vi "Tuning Model - Trial and Error.vi"() -> ()   [LabVIEW 2021]
uses:
  <vilib>/Simulation/Scripting/Companion Diagram/SimConfigNode/SimParams.ctl
  <vilib>/Simulation/Scripting/Companion Diagram/SimConfigNode/_simSolvers.ctl
  <vilib>/Simulation/Implementation/Shared/SIMSCR Execution Mode.ctl
  <vilib>/Simulation/Param Hierarchy/Typedefs/SIMPH Param Control Actions.ctl
  <vilib>/Simulation/Implementation/Shared/NILVSim_ParamChanged.vi
  <vilib>/Simulation/Implementation/Shared/NILVSIM_BeginStep.vi
  <vilib>/Simulation/Implementation/Shared/NILVSim_Manager.vi
  <vilib>/Utility/error.llb/Clear Errors.vi
  <vilib>/Simulation/Implementation/Shared/NILVSim_FinalizeModel.vi
  <vilib>/Simulation/Implementation/Shared/SIM Unbundle Sim Info.vi
  <vilib>/Simulation/Implementation/Shared/NILVSim_Initialize.vi
  <vilib>/Simulation/Utility/Implementation/NILVSim Get Time and IsAcceptedStep.vi
  <vilib>/Simulation/Implementation/Shared/SIMSH Read Queue.vi
  <vilib>/Simulation/Implementation/Shared/NILVSim_GetModelError.vi
  <vilib>/Simulation/Implementation/Shared/SIM Bundle Sim Info.vi
  <vilib>/Simulation/Implementation/XNodeFramework/SimXNode/SimX.xnode
  Blackbox/Air Heater Black Box Model.vi
  <vilib>/Simulation/Scripting/Companion Diagram/SimConfigNode/SimDog.xnode
  SubVIs/Air Heater Model.vi
  <vilib>/Simulation/Implementation/Shared/NI_SIM_Implementation.lvlib
panel:
  out "Error [°C]":dbl format="%.1g"
  in  "Model Parameters":T1={"T_init [C]"=21.5, "T [s]"=22.5, "K [C/V]"=3.9, "T_delay [s]"=2.1, "T_env [C]"=21.5}
  out "Model [°C]":dbl format="%.1g"
  out "Real Process [°C]":dbl format="%.1g"
  in  "Stop Button":bool
  out "Waveform Chart":T2(graph)
  in  "Control Signal [u]":dbl=1.0 format="%.1g"
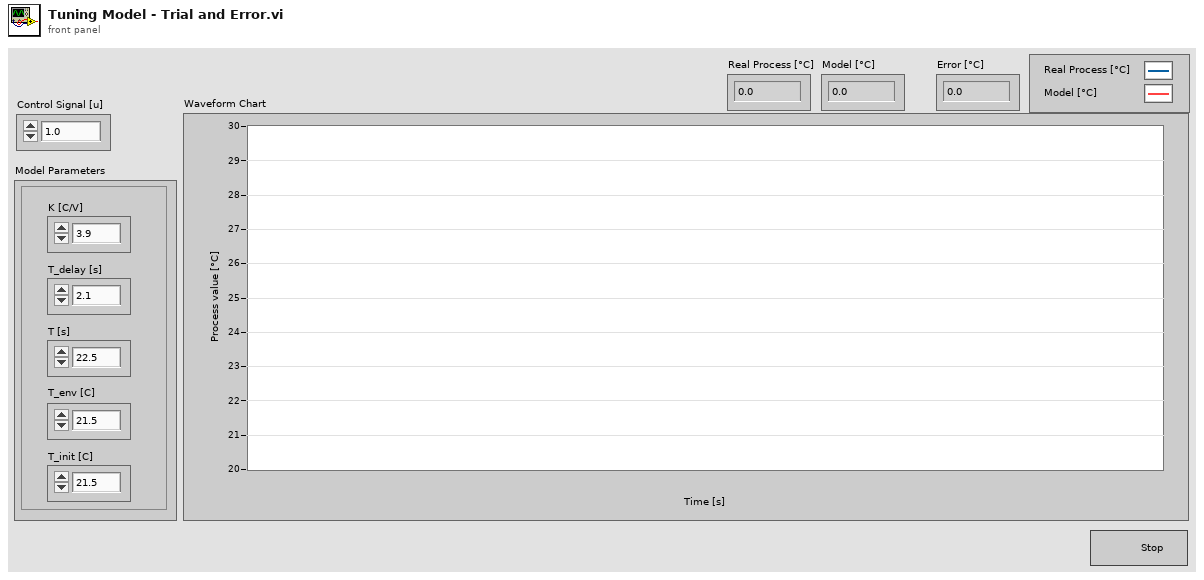
[diagram p1: front panel]
types:
  T1 = cluster{"T_init [C]":dbl, "T [s]":dbl, "K [C/V]":dbl, "T_delay [s]":dbl, "T_env [C]":dbl}
  T2 = cluster{"Output Value [20-50degC]":dbl, "Tout [C]":dbl}
  T3 = cluster{"Output Value [20-50degC]":dbl, "Tout [C]":dbl}[]
  T4 = enum16{"Simulate to Completion", "Single Time-Step Simulation (Fixed Step Only)"}
  T5 = typedef "SIMSCR Execution Mode.ctl" = enum16{"Simulate to Completion", "Single Time-Step Simulation (Fixed Step Only)"}
  T6 = typedef "SIMPH Param Control Actions.ctl" = enum16{"get params", "set params"}
  T7 = cluster{"SIMSH Sim Time":dbl, "lower limit":dbl, "Integrator":cluster{"output":dbl}, "Multiplication":cluster{"Result":dbl}, "Summation":cluster{"Result":dbl}, "Multiplication 2":cluster{"Result":dbl}, "Transport Delay":cluster{"output":dbl}, "Summation 2":cluster{"Result":dbl}}
  T8 = typedef "SimParams.ctl" = cluster{"Initial Time (s)":dbl, "Final Time (s)":dbl, "Step Size (s)":dbl, "ODE Solver":T9, "Minimum Step Size (s)":dbl, "Maximum Step Size (s)":dbl, "Relative Tolerance":dbl, "Absolute Tolerance":dbl, "Software Timing":bool, "Initial Step Size (s)":dbl, "Automatic Fixed Step Size?":bool, "Automatic Discrete Step Size?":bool, "Discrete Step Size (s)":dbl, "Calculate using Time Step":bool, "Solver Wired?":bool, "Prev.Frm.Expected End":u64, "Prev.Frm.Actual End":u64, "Prev.Frm.Finished Late?":bool, "Prev.Iter.Expected End":u64, "Prev.Iter.Actual End":u64, "Prev.Iter.Finished Late?":bool, "Expected Iteration Start":u64, "Actual Iteration Start":u64, "Expected Frame Start":u64, "Actual Frame Start":u64, "Source Name":string, "Name":string, "Period":i64, "Deadline":i64, "Offset":i64, "Start":i64, "Priority":i32, "Timeout":i32, "Processor":i32, "Mode":enum32{"No Change", "Process missed periods, maintain original phase", "Discard missed periods, maintain original phase", "Process missed periods, ignore original phase", "Discard missed periods, ignore original phase"}, "Wakeup reason":enum32{"Normal", "Aborted", "Asynchronous wakeup", "Timing source error", "Timed loop error", "Timeout"}, "Error":errorcluster, "Source Type":string, "Secondary Source Type":string, "Global End Time":u64, "Global Start Time":u64, "Full Solver Reset":bool, "Execution Mode":T5, "Nan/Inf Check":bool, "Custom Solver Library":string, "Solver Is Variable":bool, "custom solver name":string, "Signal Collection Decimation":u32}
  T9 = typedef "_simSolvers.ctl" = enum16{"Runge-Kutta 1 (Euler)", "Runge-Kutta 2", "Runge-Kutta 3", "Runge-Kutta 4", "Runge-Kutta 23 (variable)", "Runge-Kutta 45 (variable)", "BDF (variable)", "Adams-Moulton (variable)", "Rosenbrock (variable)", "Discrete States Only", "SDIRK 4 (variable)", "Radau 5 (variable)", "Radau 9 (variable)", "Radau 13 (variable)", "Radau [Variable Order] (variable)", "Gear's Method (variable)", "Linearizer", "State Query", "Trim Eval", "Custom Solver"}
  T10 = cluster{"SIMSH Sim Time":dbl, "Linear Scaling with Points.vi 2":cluster{"Output":dbl}, "Select":cluster{"s? t:f":dbl}, "Summation 3":cluster{"Result":dbl}, "Square Root":cluster{"sqrt(x)":dbl}, "Gaussian White Noise PtByPt.vi":cluster{"Gaussian white noise":dbl}, "Integrator":cluster{"output":dbl}, "Multiplication":cluster{"Result":dbl}, "Summation":cluster{"Result":dbl}, "Multiplication 2":cluster{"Result":dbl}, "Transport Delay":cluster{"output":dbl}, "Summation 2":cluster{"Result":dbl}}
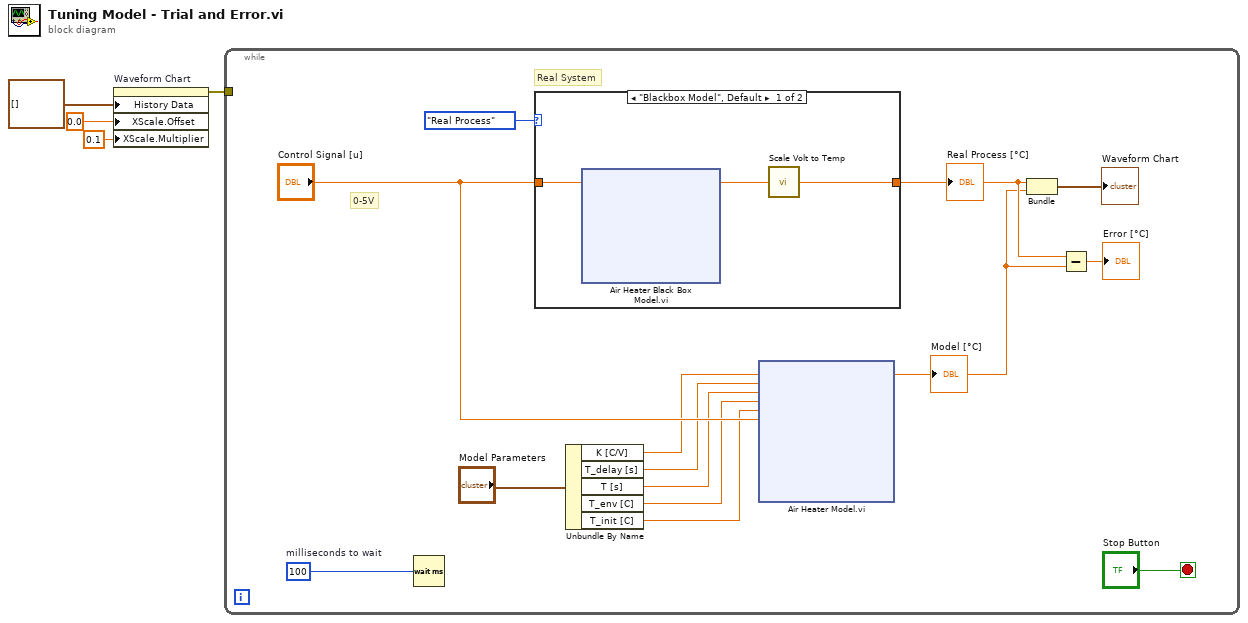
[diagram p0: block diagram]
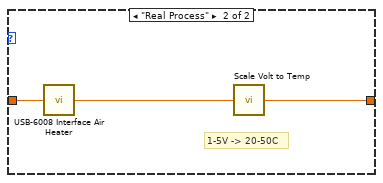
[diagram p2: hidden frame]
diagram:
  n1 = property on="Waveform Chart" class="WFChart (strict)"("History Data"=T3 [], "XScale.Offset"=0.0 ("X Scale.Offset and Multiplier:Offset"), "XScale.Multiplier"=0.1 ("X Scale.Offset and Multiplier:Multiplier")) -> (error out=w4:errorcluster)  [unwired: 2 in, 1 out]
  n2 = while {
    tunnel: w4 -> [_]
    stop <- "Stop Button" stop-if-true
    w17 = u32 100  # milliseconds to wait
    # "Real System"
    # "0-5V"
    n3 = Wait (ms)(milliseconds to wait=w17) -> ()  [unwired: 1 out]
    n4 = case shown="\"Blackbox Model\", Default" enum16{"Blackbox Model", "Real Process"}."Real Process" ("Enum") {
      tunnel: "Control Signal [u]" -> [w293 w541]
      tunnel: [w291 w539] -> w6
      frame "Blackbox Model", Default {
        n5 = xnode "Air Heater Black Box Model.vi"("Control Signal [0-5V]"=w293) -> ("Tout [1-5V]"=w292:dbl)  [unwired: 2 in, 1 out]
        n6 = call "Scale Volt to Temp.vi"("Input Value [1-5V]"=w292) -> ("Output Value [20-50degC]"=w291:dbl)
      }
      frame "Real Process" {
        # "1-5V -> 20-50C"
        n7 = call "USB-6008 Interface Air Heater.vi"("Control Signal [0-5V]"=w541) -> ("Process Value [1-5V]"=w540:dbl)
        n8 = call "Scale Volt to Temp.vi"("Input Value [1-5V]"=w540) -> ("Output Value [20-50degC]"=w539:dbl)
      }
    }
    "Real Process [°C]" <- w6
    n9 = Unbundle By Name("Model Parameters") -> ("K [C/V]"=w12:dbl, "T_delay [s]"=w11:dbl, "T [s]"=w10:dbl, "T_env [C]"=w9:dbl, "T_init [C]"=w8:dbl)
    n10 = xnode "Air Heater Model.vi"("K [C/V]"=w12, "T_delay [s]"=w11, "T [s]"=w10, "T_env [C]"=w9, "T_init [C]"=w8, "u [V]"="Control Signal [u]") -> ("Tout [C]"=w5:dbl)  [unwired: 2 in, 10 out]
    "Model [°C]" <- w5
    n11 = Bundle("Output Value [20-50degC]"=w6, "Tout [C]"=w5) -> (→"Waveform Chart":T2)  [unwired: 1 in]
    n12 = Subtract(x=w6, y=w5) -> (x-y=→"Error [°C]":dbl)
  }
